vi "Controller Read Inputs.vi"(8 "error in (no error)":errorcluster, 9 "PS Status Variables":refnum<k21>[](array[refnum]), 10 "PS Reading Variables":refnum<k21>[](array[refnum]), 11 "BPM Variables":refnum<k21>[](array[refnum])) -> (0 "error out":errorcluster, 1 "PS Status (per PS Rack)":u8[](array[numeric]), 2 "PS Readings":dbl[](array[numeric]), 3 "BPM Readings":dbl[](array[numeric]))   [LabVIEW 2011, in "Controller VIs.lvlib"]
doc: "Read all input variables from the Acquisition and Actuation chassis."
uses:
  Controller VIs.lvlib
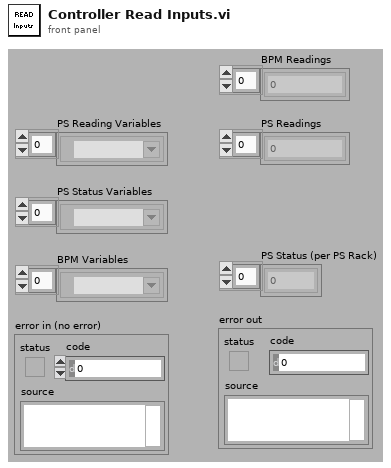
[diagram p1: front panel]
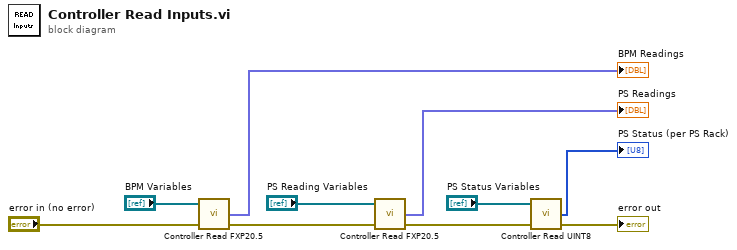
[diagram p0: block diagram]
diagram:
  n1 = call "Controller Read FXP20.5.vi"("error in (no error)"="error in (no error)", "Variables"="BPM Variables") -> ("error out"=w3:errorcluster, "Values"=→"BPM Readings":fxp<+/-,20,5>[])  [unwired: 2 in]
  n2 = call "Controller Read FXP20.5.vi"("error in (no error)"=w3, "Variables"="PS Reading Variables") -> ("error out"=w2:errorcluster, "Values"=→"PS Readings":fxp<+/-,20,5>[])  [unwired: 2 in]
  n3 = call "Controller Read UINT8.vi"("error in (no error)"=w2, "Variables"="PS Status Variables") -> ("error out"=→"error out":errorcluster, "Values"=→"PS Status (per PS Rack)":u8[])  [unwired: 2 in]
